vi "MPU.vi"(1 "DebugOut":refnum<k21>, 2 "error in (no error)":errorcluster, 3 "cRIO I/O Device":refnum<k21>, 4 "FIFO":refnum<k21>) -> (0 "error out":errorcluster)   [LabVIEW 2018, in "Modbus_Processing_Unit.lvlib"]
uses:
  Modbus_Processing_Unit.lvlib
  <vilib>/rvi/Emulation/niFpgaGetClockAttributes.vi
  <vilib>/rvi/Emulation/niFpgaSctlEmulationGetInTimedLoop.vi
  <vilib>/rvi/Emulation/niFpgaEmulationReportErrorSimple.vi
  <vilib>/rvi/DataTransferAndStorage/Container/Common/niFpgaContainerExecOnDevCompGetState.vi
  <vilib>/rvi/Emulation/niFpgaEmulationIsFPGAContextNoSignature.vi
  <vilib>/rvi/errors/niFpgaSetErrorForExecOnDevCompSimple.vi
  <vilib>/rvi/eio/common/nirviEmuReportErrorAndStop.vi
  <vilib>/rvi/DataTransferAndStorage/Container/Common/niFpgaContainerGetUniqueNameForEmu.vi
  <vilib>/rvi/FIFO/Fifo_Resource/nirvififoEmulationSetSize.vi
  <vilib>/rvi/FIFO/Fifo_Resource/nirviFifoEmulationQueueMgr.vi
  <instcachedir>/0/nirviFifoEmulationQueueMgr_E5CAEC123FF24DC58D834DCA3CDAA9B5.lvgen/nirviFifoEmulationQueueMgr_E5CAEC123FF24DC58D834DCA3CDAA9B5_001.vi
  <vilib>/rvi/FIFO/Fifo_Resource/nirvififoEmulationDetermineInputValidOut.vi
  <vilib>/rvi/FIFO/Fifo_Resource/nirvififoEmulationCreateLock.vi
  <vilib>/rvi/Emulation/niFpgaProcessEmulError.vi
  <vilib>/rvi/FIFO/Fifo_Resource/nirvififoEmulationObtainLock.vi
  <vilib>/rvi/FIFO/Fifo_Resource/nirvififoEmulationReleaseLock.vi
  <vilib>/rvi/occurrence/nirviWaitOnOccurrenceBase.vi
  <vilib>/rvi/errors/nirviReportUnexpectedCaseInternalError.vi
  <vilib>/rvi/errors/nirviReportUnexpectedCaseInternalError (U32).vi
  <vilib>/Utility/error.llb/Clear Errors.vi
  <vilib>/rvi/interface/RandomDataEmulation/niFpgaRandomDataHandleErrors.vi
  <vilib>/rvi/eio/common/nirviEmuTemplateMethod_errors.vi
  <vilib>/rvi/Emulation/niFpgaCriticalErrorInLSC.vi
  <vilib>/rvi/DataTransferAndStorage/Container/XNode/niFpgaContainer.xnode
  <vilib>/rvi/FIFO/Fifo_Resource/niFpgaFifoEmulationRefIn.vi
  <vilib>/eio/EIOMethodNode/EIOMethodNode.xnode
panel:
  out "Output":u8[](array[numeric])
  in  "IP":i16
  in  "Instructions":u8[](array[numeric])=[0, 0, 0, 0, 0, 0, 0, 0, 0, 0, 0, 0, 0, 0, 0, 0, 0, 0, 0, 0, 0, 0, 0, 0, 0, 0, 0, 0, 0, 0, 0, 0, 0, 0, 0, 0, 0, 0, 0, 0, 0, 0, 0, 0, 0, 0, 0, 0, 0, 0, 0, 0, 0, 0, 0, 0, 0, 0, 0, 0, 0, 0, 0, 0, 0, 0, 0, 0, 0, 0, 0, 0, 0, 0, 0, 0, 0, 0, 0, 0, 0, 0, 0, 0, 0, 0, 0, 0, 0, 0, 0, 0, 0, 0, 0, 0, 0, 0, 0, 0]
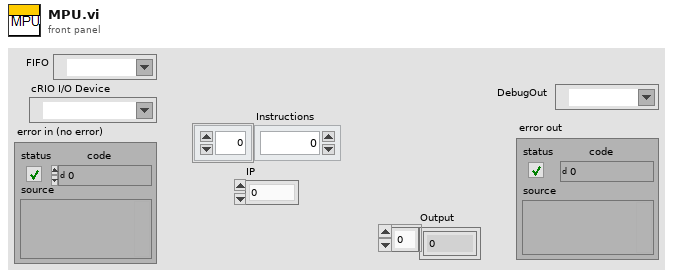
[diagram p1: front panel]
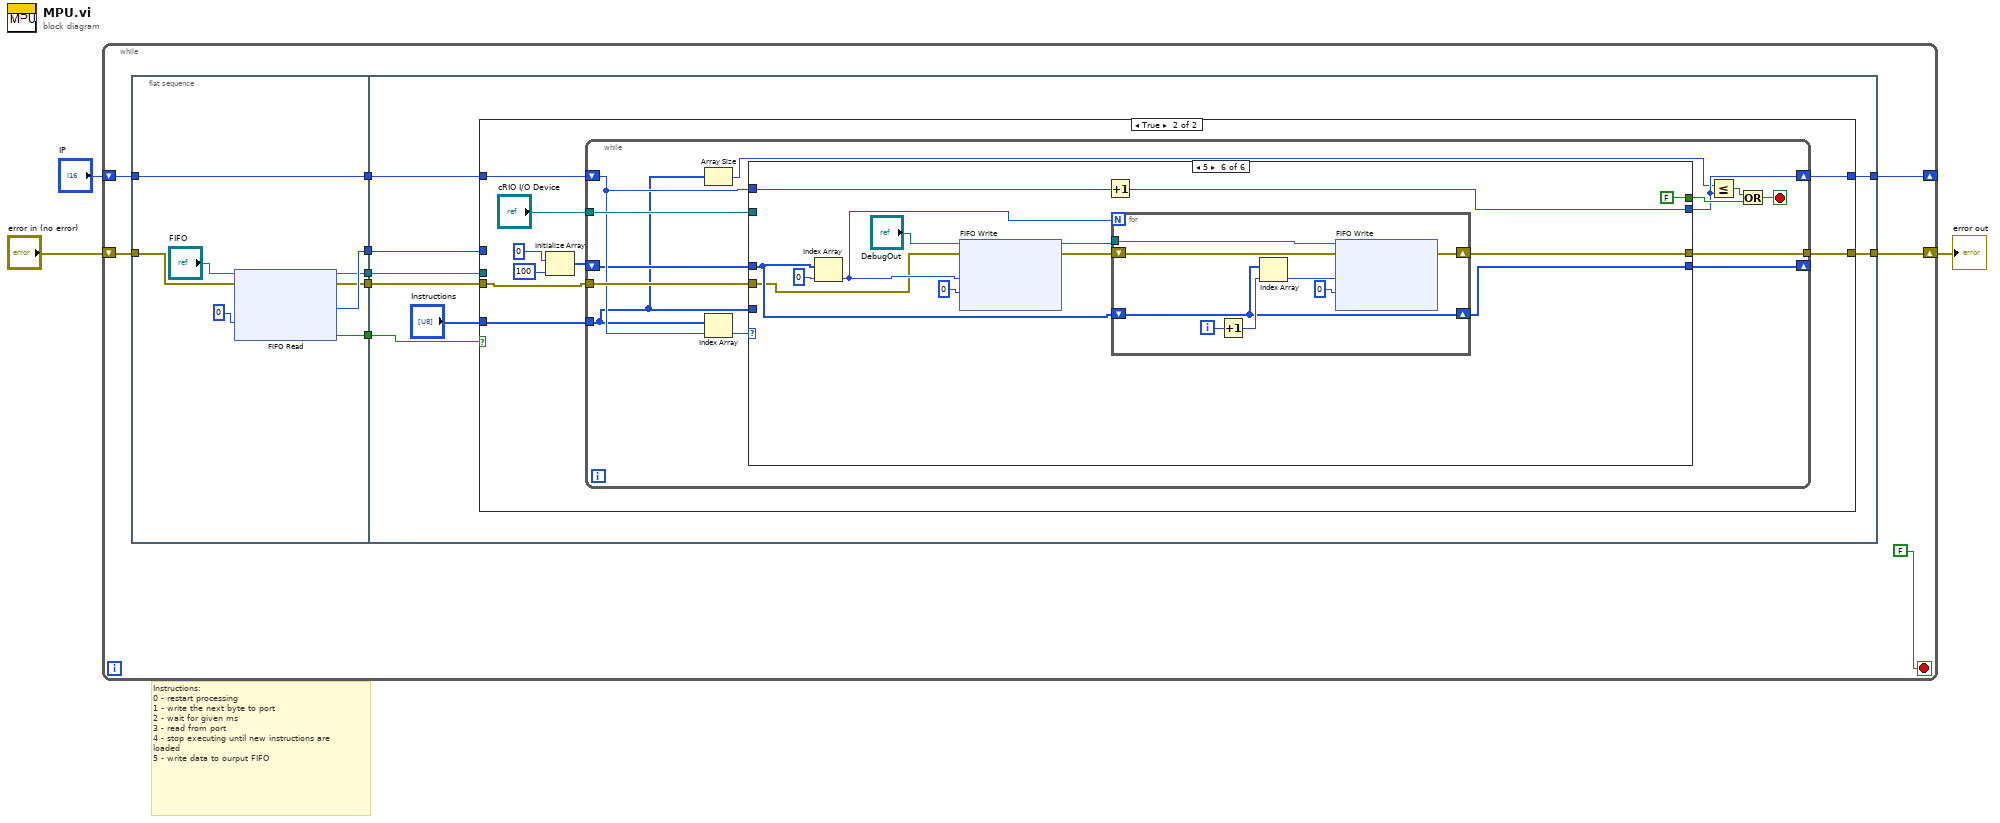
[diagram p0: block diagram]
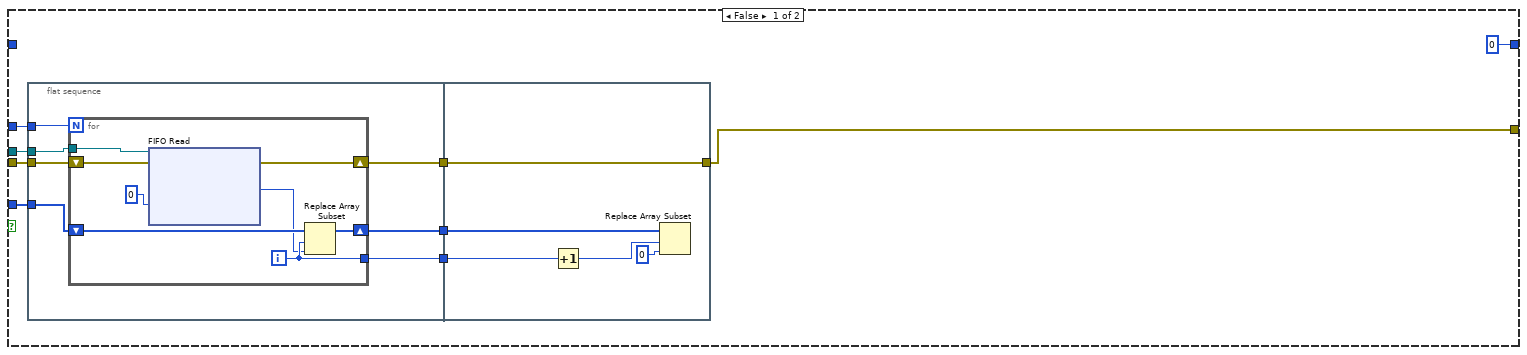
[diagram p2: hidden frame]
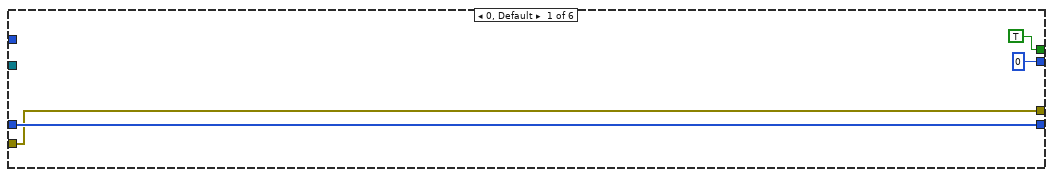
[diagram p3: hidden frame]
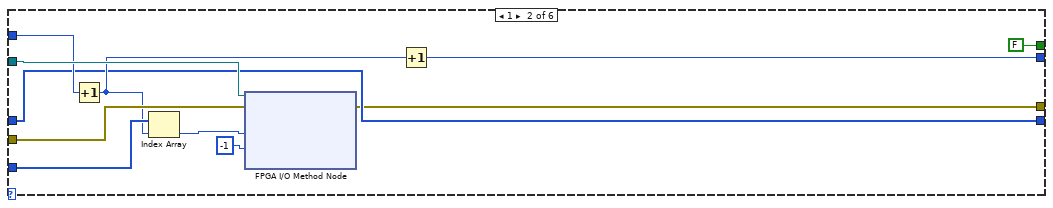
[diagram p4: hidden frame]
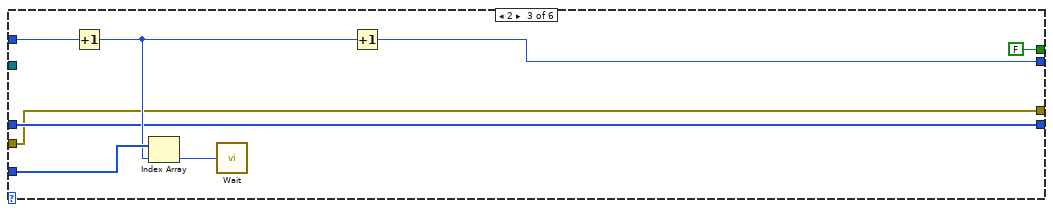
[diagram p5: hidden frame]
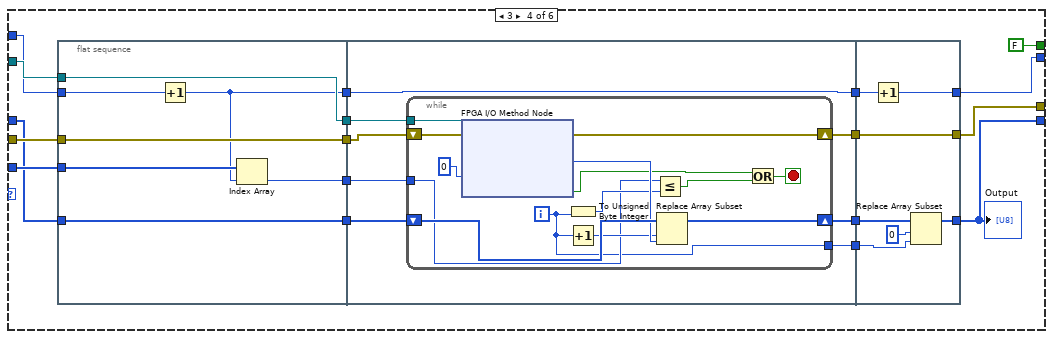
[diagram p6: hidden frame]
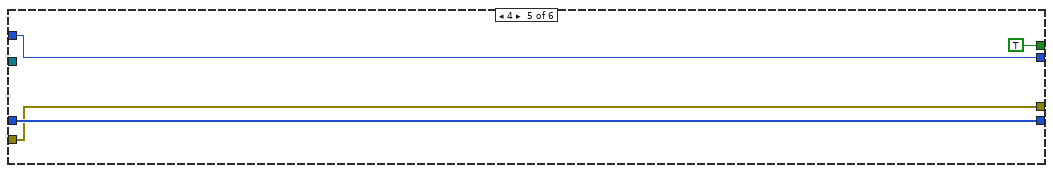
[diagram p7: hidden frame]
diagram:
  # "Instructions:\n0 - restart processing\n1 - write the next byte to port\n2 - wait for given ms\n3 - read from port\n4 - stop executing until new instructions are loaded\n5 - write data to ourput FIFO"
  n1 = while {
    shift-right: [w4] -> w2
    shift-left: "error in (no error)" -> [w13]
    shift-right: [w5] -> _
    shift-left: "IP" -> [w7]
    stop <- FALSE stop-if-true
    n2 = flat-sequence {
      tunnel: w13 -> [w21]
      tunnel: [w20] -> w12
      tunnel: [w19] -> w11
      tunnel: [w18] -> w10
      tunnel: [w16] -> w9
      tunnel: w7 -> [w14]
      tunnel: [w14] -> w6
      tunnel: w12 -> [w28]
      tunnel: w11 -> [w27]
      tunnel: w10 -> [w26]
      tunnel: w9 -> [w25]
      tunnel: w6 -> [w24]
      tunnel: [w23] -> w5
      tunnel: [w22] -> w4
      frame #0 {
        n3 = xnode ("FIFO Read")("Timeout"=0, "error in (no error)"=w21, "FIFO In"="FIFO") -> ("Element"=w20:u8, "Timed Out?"=w19:bool, "error out"=w18:errorcluster, "FIFO Out"=w16:refnum<k21>)
      }
      frame #1 {
        n4 = case shown="True" w27 {
          tunnel: w26 -> [w38 w66]
          tunnel: w28 -> [w37 _]
          tunnel: "Instructions" -> [w36 w67]
          tunnel: w25 -> [w32 _]
          tunnel: w24 -> [_ w64]
          tunnel: [i16 0 ("IP") w63] -> w23
          tunnel: [w30 w59] -> w22
          frame False {
            n5 = flat-sequence {
              tunnel: w36 -> [w42]
              tunnel: w37 -> [w43]
              tunnel: w38 -> [w45]
              tunnel: [w44] -> w35
              tunnel: [w41] -> w34
              tunnel: [w40] -> w33
              tunnel: w32 -> [w39]
              tunnel: [w58] -> w30
              tunnel: w35 -> [w58]
              tunnel: w34 -> [w57]
              tunnel: w33 -> [w56]
              frame #0 {
                n6 = for {
                  N: w43 -> [_]
                  shift-right: [w52] -> w44
                  shift-left: w45 -> [w53]
                  shift-right: [w49] -> w41
                  shift-left: w42 -> [w51]
                  tunnel: [w48] -> w40
                  tunnel: w39 -> [w47]
                  i -> [w48]
                  n7 = xnode ("FIFO Read")("Timeout"=0, "error in (no error)"=w53, "FIFO In"=w47) -> ("Element"=w46:u8, "error out"=w52:errorcluster)  [unwired: 2 out]
                  n8 = Replace Array Subset(array=w51, new element=w46, index=w48) -> (w49:u8[])
                }
              }
              frame #1 {
                n9 = Increment(x=w56) -> (x+1=w55:i32)
                n10 = Replace Array Subset(array=w57, new element=u8 0 ("new element/subarray"), index=w55) -> ()  [unwired: 1 out]
              }
            }
          }
          frame True {
            n11 = Initialize Array(u8 0 ("element"), 100 ("dimension size")) -> (w60:u8[])
            n12 = while {
              tunnel: w67 -> [w73]
              tunnel: "cRIO I/O Device" -> [w79]
              tunnel: w66 -> [w78]
              shift-right: [w70] -> w63
              shift-left: w64 -> [w76]
              shift-right: [w74] -> _
              shift-left: w60 -> [w75]
              tunnel: [w68] -> w59
              stop <- w72 stop-if-true
              n13 = Array Size(array=w73) -> (size(s)=w69:i32)
              n14 = Index Array(array=w73, index=w76) -> (element=w77:u8)
              n15 = case shown="5" w77 {
                tunnel: [TRUE FALSE FALSE FALSE TRUE FALSE] -> w80
                tunnel: w79 -> [_ w93 _ w114 _ _]
                tunnel: w78 -> [w81 w94 w96 w115 w158 w164]
                tunnel: w76 -> [_ w89 w101 w111 w160 w169]
                tunnel: [i16 0 w87 w100 w120 w160 w168] -> w70
                tunnel: w73 -> [_ w91 w103 w121 _ _]
                tunnel: [w82 w86 w97 w107 w159 w171] -> w74
                tunnel: w75 -> [w82 w86 w97 w106 w159 w172]
                tunnel: [w81 w85 w96 w104 w158 w167] -> w68
                frame 0, Default {
                }
                frame 1 {
                  n16 = Increment(x=w89) -> (x+1=w88:i16)
                  n17 = Index Array(array=w91, index=w88) -> (element=w90:u8)
                  n18 = xnode "FPGA I/O Method Node"("error in"=w94, "FPGA I/O In"=w93, "Data"=w90, "Timeout (ms)"=-1) -> ("error out"=w85:errorcluster)  [unwired: 2 out]
                  n19 = Increment(x=w88) -> (x+1=w87:i16)
                }
                frame 2 {
                  n20 = Increment(x=w101) -> (x+1=w99:i16)
                  n21 = Index Array(array=w103, index=w99) -> (element=w102:u8)
                  n22 = call "Wait"("Count(mSec)"=w102) -> ()  [unwired: 1 out]
                  n23 = Increment(x=w99) -> (x+1=w100:i16)
                }
                frame 3 {
                  n24 = flat-sequence {
                    tunnel: w121 -> [w128]
                    tunnel: [w127] -> w117
                    tunnel: w115 -> [w126]
                    tunnel: [w126] -> w116
                    tunnel: w114 -> [w125]
                    tunnel: [w125] -> w113
                    tunnel: w111 -> [w124]
                    tunnel: [w123] -> w110
                    tunnel: w106 -> [w122]
                    tunnel: [w122] -> w105
                    tunnel: [w136] -> w119
                    tunnel: [w135] -> w118
                    tunnel: w117 -> [w131]
                    tunnel: w116 -> [w134]
                    tunnel: w113 -> [w133]
                    tunnel: [w132] -> w112
                    tunnel: w110 -> [w136]
                    tunnel: [w130] -> w108
                    tunnel: w105 -> [w129]
                    tunnel: [w156] -> w104
                    tunnel: [w155] -> w120
                    tunnel: w119 -> [w157]
                    tunnel: w118 -> [w156]
                    tunnel: w112 -> [w154]
                    tunnel: [w153] -> w107
                    tunnel: w108 -> [w152]
                    frame #0 {
                      n25 = Increment(x=w124) -> (x+1=w123:i16)
                      n26 = Index Array(array=w128, index=w123) -> (element=w127:u8)
                    }
                    frame #1 {
                      n27 = while {
                        shift-right: [w149] -> w135
                        shift-left: w134 -> [w150]
                        shift-right: [w148] -> w132
                        shift-left: w129 -> [w147]
                        tunnel: w133 -> [w146]
                        tunnel: w131 -> [w140]
                        tunnel: [w139] -> w130
                        i -> [w139]
                        stop <- w142 stop-if-true
                        n28 = xnode "FPGA I/O Method Node"("error in"=w150, "FPGA I/O In"=w146, "Timeout (ms)"=0) -> ("error out"=w149:errorcluster, "Data"=w145:u8, "Timed Out"=w138:bool)  [unwired: 1 out]
                        n29 = To Unsigned Byte Integer(number=w139) -> (unsigned 8bit integer=w141:u8)
                        n30 = Increment(x=w139) -> (x+1=w143:i32)
                        n31 = Less Or Equal?(x=w140, y=w141) -> (x <= y?=w137:bool)
                        n32 = Replace Array Subset(array=w147, new element=w145, index=w143) -> (w148:u8[])
                        n33 = Or(x=w138, y=w137) -> (x .or. y?=w142:bool)
                      }
                    }
                    frame #2 {
                      n34 = Increment(x=w157) -> (x+1=w155:i16)
                      n35 = Replace Array Subset(array=w154, new element=w152, index=0) -> (w153:u8[])
                    }
                  }
                  "Output" <- w107
                }
                frame 4 {
                }
                frame 5 {
                  n36 = Index Array(array=w172, index=0) -> (element=w165:u8)
                  n37 = xnode "FIFO Write"("Element"=w165, "Timeout"=0, "error in (no error)"=w164, "FIFO In"="DebugOut") -> ("error out"=w163:errorcluster, "FIFO Out"=w166:refnum<k21>)  [unwired: 1 out]
                  n38 = Increment(x=w169) -> (x+1=w168:i16)
                  n39 = for {
                    N: w165 -> [_]
                    shift-right: [w180] -> w171
                    shift-left: w172 -> [w180]
                    tunnel: w166 -> [w179]
                    shift-right: [w175] -> w167
                    shift-left: w163 -> [w178]
                    i -> [w182]
                    n40 = Increment(x=w182) -> (x+1=w181:i32)
                    n41 = Index Array(array=w180, index=w181) -> (element=w176:u8)
                    n42 = xnode "FIFO Write"("Element"=w176, "Timeout"=0, "error in (no error)"=w178, "FIFO In"=w179) -> ("error out"=w175:errorcluster)  [unwired: 2 out]
                  }
                }
              }
              n43 = Less Or Equal?(x=w69, y=w70) -> (x <= y?=w71:bool)
              n44 = Or(x=w71, y=w80) -> (x .or. y?=w72:bool)
            }
          }
        }
      }
    }
  }
  "error out" <- w2
